vi "TSCAN_GetCANDBInfo.vi"(8 "ADatabaseld":u32=1, 10 "路径输入":path) -> (0 "ID":i32[](array[numeric]) format="%x", 1 "SignalName":string[][](array[string]), 2 "Message":string[](array[string]), 3 "路径输出":path, 4 "Message&ID":string[](array[string]), 5 "ALLName":string[](array[string]))   [LabVIEW 2019]
uses:
  <vilib>/Utility/importsl/GetValueByPointer/datatype.ctl
  <vilib>/Utility/importsl/GetValueByPointer/GetValueByPointer.xnode
panel:
  out "tsdb_load_can_db 2":i32
  out "tsdb_load_can_db":i32
  # "同一行中属于相同的Mssage"
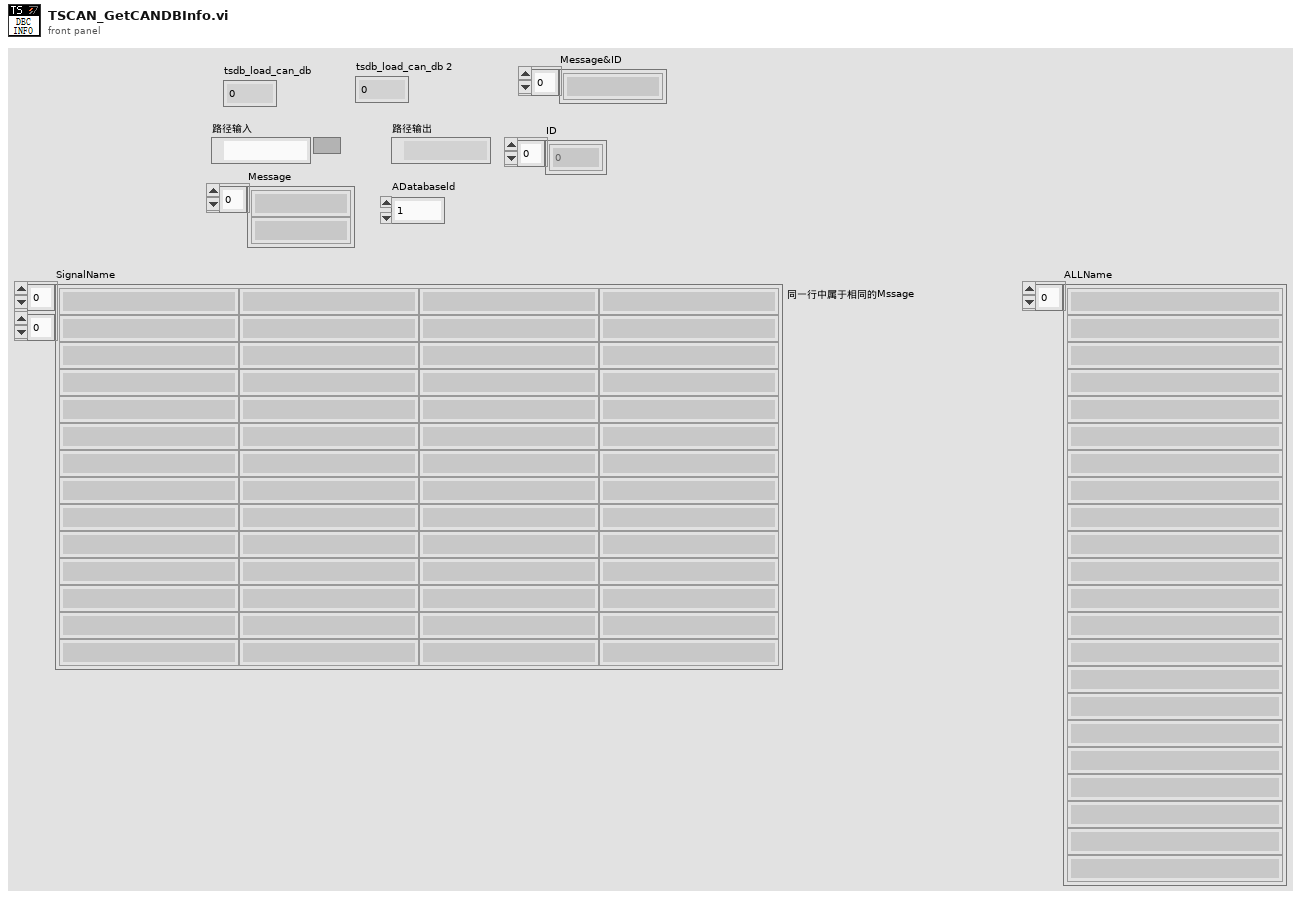
[diagram p1: front panel]
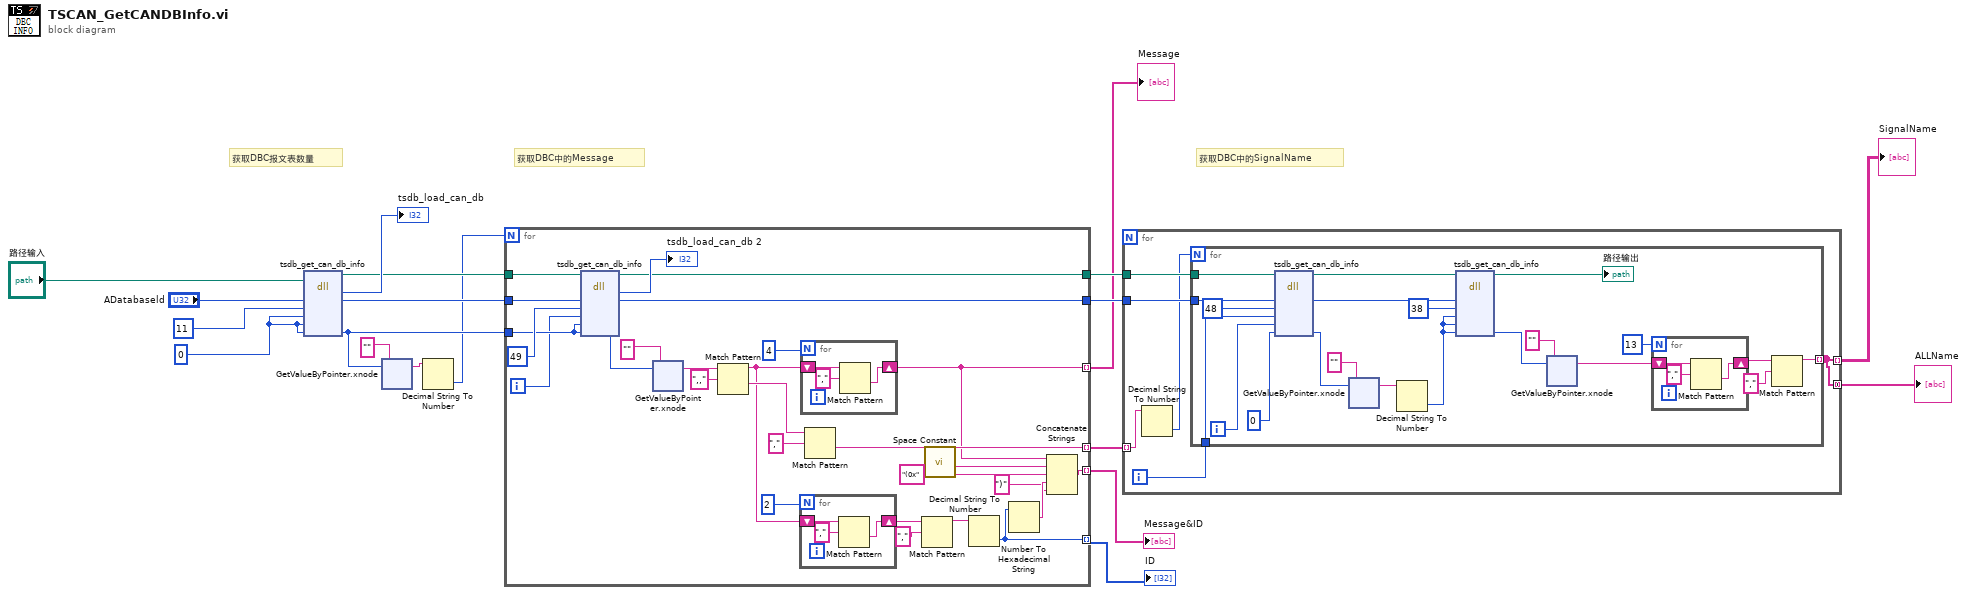
[diagram p0: block diagram]
diagram:
  w7 = u32 0 ("AIndex")
  # "获取DBC中的SignalName"
  # "获取DBC中的Message"
  # "获取DBC报文表数量"
  n1 = dll-call lib="PTH27abs EDemo同星\nTSCAN_V1.0ConfigTSMaster.dll" fn="tsdb_get_can_db_info"(path in="路径输入", "ADatabaseld"="ADatabaseld", "AType"=u32 11, "AIndex"=w7, "ASubIndex"=w7, "Return"=w7) -> (path out=w14:path, "tsdb_load_can_db"=→"tsdb_load_can_db":i32, "ADatabaseld"=w15:u32, "Return"=w13:i32)  [unwired: 5 in, 1 out]
  n2 = xnode "GetValueByPointer.xnode"("Pointer"=w13, "InputType"="" ("参数6")) -> ("Output"=w12:string)  [unwired: 2 in, 1 out]
  n3 = Decimal String To Number(string=w12) -> (number=w11:i32)  [unwired: 2 in, 1 out]
  n4 = for {
    N: w11 -> [_]
    tunnel: w15 -> [w44]
    tunnel: w14 -> [w43]
    tunnel: w13 -> [w38]
    tunnel: [w21] -> w6 mode=indexing
    tunnel: [w28] -> w10 mode=indexing
    tunnel: [w35] -> w9
    tunnel: [w34] -> w8
    tunnel: [w25] -> w3 mode=indexing
    tunnel: [w23] -> w2 mode=indexing
    i -> [w37]
    n5 = dll-call lib="PTH27abs EDemo同星\nTSCAN_V1.0ConfigTSMaster.dll" fn="tsdb_get_can_db_info"(path in=w43, "ADatabaseld"=w44, "AType"=u32 49, "AIndex"=w37, "ASubIndex"=w38, "Return"=w38) -> (path out=w35:path, "tsdb_load_can_db"=→"tsdb_load_can_db 2":i32, "ADatabaseld"=w34:u32, "Return"=w46:i32)  [unwired: 5 in, 1 out]
    n6 = xnode "GetValueByPointer.xnode"("Pointer"=w46, "InputType"="" ("参数6")) -> ("Output"=w40:string)  [unwired: 2 in, 1 out]
    n7 = Match Pattern(string=w40, regular expression=",," ("正则表达式")) -> (before substring=w31:string, after substring=w32:string)  [unwired: 1 in, 2 out]
    n8 = for {
      N: 2 -> [_]
      shift-right: [w48] -> w29
      shift-left: w31 -> [w50]
      n9 = Match Pattern(string=w50, regular expression="," ("正则表达式")) -> (after substring=w48:string)  [unwired: 1 in, 3 out]
    }
    n10 = for {
      N: 4 -> [_]
      shift-right: [w51] -> w21
      shift-left: w31 -> [w53]
      n11 = Match Pattern(string=w53, regular expression="," ("正则表达式")) -> (after substring=w51:string)  [unwired: 1 in, 3 out]
    }
    n12 = Match Pattern(string=w32, regular expression="," ("正则表达式")) -> (after substring=w28:string)  [unwired: 1 in, 3 out]
    n13 = Match Pattern(string=w29, regular expression="," ("正则表达式")) -> (before substring=w26:string)  [unwired: 1 in, 3 out]
    n14 = call <vilib>:"Space Constant.vi"() -> ("String"=w20:string)
    n15 = Decimal String To Number(string=w26) -> (number=w25:i32)  [unwired: 2 in, 1 out]
    n16 = Number To Hexadecimal String(2:w25) -> (0:w24:string)  [unwired: 1 in]
    n17 = Concatenate Strings(w21, w20, "(0x" ("字符串"), w24, ")" ("字符串")) -> (w23:string)
  }
  "Message" <- w6
  "ID" <- w3
  "Message&ID" <- w2
  n18 = for {
    tunnel: w10 -> [w69] mode=indexing
    tunnel: w9 -> [w71]
    tunnel: w8 -> [w70]
    tunnel: [w66] -> w4 mode=indexing
    tunnel: [w66] -> w1 mode=concatenating
    i -> [w67]
    n19 = Decimal String To Number(string=w69) -> (number=w68:i32)  [unwired: 2 in, 1 out]
    n20 = for {
      N: w68 -> [_]
      tunnel: w71 -> [w92]
      tunnel: w70 -> [w91]
      tunnel: [w84] -> w66 mode=indexing
      tunnel: w67 -> [w81]
      i -> [w82]
      n21 = dll-call lib="PTH27abs EDemo同星\nTSCAN_V1.0ConfigTSMaster.dll" fn="tsdb_get_can_db_info"(path in=w92, "ADatabaseld"=w91, "AType"=u32 48, "AIndex"=w81, "ASubIndex"=w82, "Return"=u32 0 ("ASubIndex")) -> (path out=w79:path, "ADatabaseld"=w78:u32, "Return"=w88:i32)  [unwired: 6 in, 1 out]
      n22 = xnode "GetValueByPointer.xnode"("Pointer"=w88, "InputType"="" ("参数6")) -> ("Output"=w80:string)  [unwired: 2 in, 1 out]
      n23 = Decimal String To Number(string=w80) -> (number=w76:i32)  [unwired: 2 in, 1 out]
      n24 = dll-call lib="PTH27abs EDemo同星\nTSCAN_V1.0ConfigTSMaster.dll" fn="tsdb_get_can_db_info"(path in=w79, "ADatabaseld"=w78, "AType"=u32 38, "AIndex"=w76, "ASubIndex"=w76, "Return"=w76) -> (path out=→"路径输出":path, "Return"=w73:i32)  [unwired: 7 in, 1 out]
      n25 = xnode "GetValueByPointer.xnode"("Pointer"=w73, "InputType"="" ("参数6")) -> ("Output"=w72:string)  [unwired: 2 in, 1 out]
      n26 = for {
        N: 13 -> [_]
        shift-right: [w105] -> w86
        shift-left: w72 -> [w107]
        n27 = Match Pattern(string=w107, regular expression="," ("正则表达式")) -> (after substring=w105:string)  [unwired: 1 in, 3 out]
      }
      n28 = Match Pattern(string=w86, regular expression="," ("正则表达式")) -> (before substring=w84:string)  [unwired: 1 in, 3 out]
    }
  }
  "SignalName" <- w4
  "ALLName" <- w1
